vi "Main.vi"   [LabVIEW 2019, in "ModuleE.lvlib"]
uses:
  ModuleE.lvlib
  ModuleD/ModuleD.lvclass
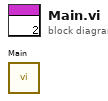
[diagram p0: block diagram]
diagram:
  n1 = call "Main.vi"() -> ()  [unwired: 12 in]
